vi "SEK2020v1SubVIOdometria.vi"(4 "Distância na horizontal":dbl=5.0 format="%#_13g", 6 "NXT/EV3":T1) -> (0 "Distância na vertical":dbl, 2 "NXT/EV3 2":T1)   [LabVIEW 2016]
uses:
  <vilib>/NXT/Subs/LVHSConnector.ctl
  <vilib>/NXT/LegoClasses/BrickReference/BrickReference.lvclass
  <vilib>/NXT/Block Support/NXT_OutputPort.ctl
  <vilib>/NXT/Block Support/NXT_InputPort.ctl
  <vilib>/NXT/Dual Mode Library/Sensors/EV3_Gyro_Reset.vi
  <vilib>/NXT/Dual Mode Library/Motors/ResetMotor.vi
  <vilib>/NXT/Dual Mode Library/Sensors/EV3_Gyro_Angle.vi
  <vilib>/NXT/NXTIO Xnodes/NXTIONodeSubVIs/NXTMoveMotors.vi
  <vilib>/NXT/Dual Mode Library/Motors/Rotation.vi
  <vilib>/NXT/NXTIO Xnodes/AddressXNode/NXTIOAddress.xnode
  <vilib>/NXT/NXTIO Xnodes/NXTIOXNode/NXTIO.xnode
panel:
  in  "Kp":dbl format="%#_13g"
  in  "K1":dbl
  in  "K2":dbl
  out "Dl":dbl
  out "Dr":dbl
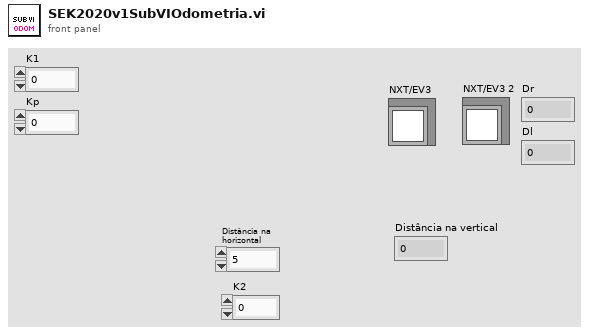
[diagram p1: front panel]
types:
  T1 = typedef "LVHSConnector.ctl" = refnum<class "BrickReference.lvclass">
  T2 = typedef "NXT_InputPort.ctl" = u32
  T3 = typedef "NXT_OutputPort.ctl" = u8
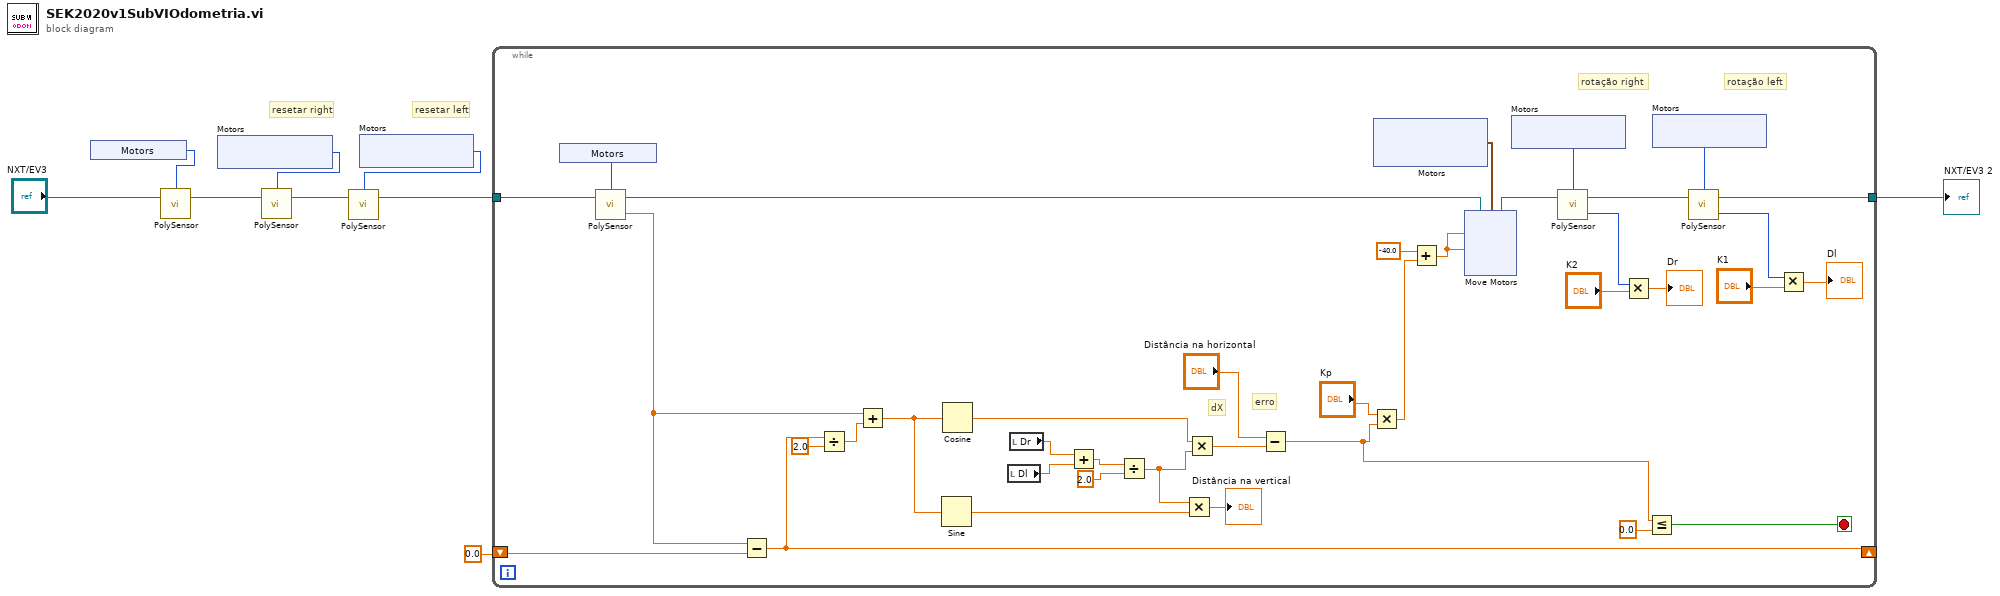
[diagram p0: block diagram]
diagram:
  # "resetar left"
  # "resetar right"
  n1 = xnode "Motors"() -> ("Sensor"=w2:T2)
  n2 = call-poly <vilib>:"PolySensor.vi"("NXT/EV3"="NXT/EV3", "Port (Port 1)"=w2) -> ("NXT/EV3"=w4:T1)  [unwired: 2 in]
  n3 = xnode "Motors"() -> ("Motor"=w8:T3)
  n4 = call-poly <vilib>:"PolySensor.vi"("NXT/EV3"=w4, "Port (All Ports)"=w8) -> ("NXT/EV3"=w7:T1)  [unwired: 2 in]
  n5 = xnode "Motors"() -> ("Motor"=w5:T3)
  n6 = call-poly <vilib>:"PolySensor.vi"("NXT/EV3"=w7, "Port (All Ports)"=w5) -> ("NXT/EV3"=w6:T1)  [unwired: 2 in]
  n7 = while {
    tunnel: w6 -> [w34]
    tunnel: [w42] -> w9
    shift-right: [w32] -> _
    shift-left: sgl 0.0 -> [w33]
    stop <- w16 stop-if-true
    # "erro"
    # "dX"
    # "rotação left"
    # "rotação right"
    n8 = xnode "Motors"() -> ("Sensor"=w44:T2)
    n9 = call-poly <vilib>:"PolySensor.vi"("NXT/EV3"=w34, "Port (Port 1)"=w44) -> ("Degrees"=w30:sgl, "NXT/EV3"=w43:T1)  [unwired: 1 in]
    n10 = Subtract(x=w30, y=w33) -> (x-y=w32:sgl)
    n11 = Divide(x=w32, y=sgl 2.0) -> (x/y=w29:sgl)
    n12 = Add(x=w30, y=w29) -> (x+y=w13:sgl)
    n13 = Sine(x=w13) -> (sin(x)=w12:sgl)
    n14 = Cosine(x=w13) -> (cos(x)=w23:sgl)
    n15 = local read "Dl"() -> (w26:dbl)
    n16 = local read "Dr"() -> (w27:dbl)
    n17 = Add(x=w27, y=w26) -> (x+y=w25:dbl)
    n18 = Divide(x=w25, y=2.0) -> (x/y=w11:dbl)
    n19 = Multiply(x=w11, y=w12) -> (x*y=→"Distância na vertical":dbl)
    n20 = Multiply(x=w23, y=w11) -> (x*y=w22:dbl)
    n21 = Subtract(x="Distância na horizontal", y=w22) -> (x-y=w15:dbl)
    n22 = Multiply(x="Kp", y=w15) -> (x*y=w19:dbl)
    n23 = xnode "Motors"() -> ("Motor"=w47:cluster{"Port":T3, "Port":T3})
    n24 = Add(x=-40.0, y=w19) -> (x+y=w17:dbl)
    n25 = xnode "Move Motors"("Power/Speed 2"=w17, "Power/Speed 1"=w17, "Motors"=w47, "NXT/EV3"=w43) -> ("NXT/EV3"=w46:T1)
    n26 = xnode "Motors"() -> ("Motor"=w41:T3)
    n27 = call-poly <vilib>:"PolySensor.vi"("NXT/EV3"=w46, "Port (Port A)"=w41) -> ("Angle of Rotation"=w39:i32, "NXT/EV3"=w45:T1)  [unwired: 1 in]
    n28 = Multiply(x=w39, y="K2") -> (x*y=→"Dr":dbl)
    n29 = Less Or Equal?(x=w15, y=0.0) -> (x <= y?=w16:bool)
    n30 = xnode "Motors"() -> ("Motor"=w40:T3)
    n31 = call-poly <vilib>:"PolySensor.vi"("NXT/EV3"=w45, "Port (Port A)"=w40) -> ("Angle of Rotation"=w37:i32, "NXT/EV3"=w42:T1)  [unwired: 1 in]
    n32 = Multiply(x=w37, y="K1") -> (x*y=→"Dl":dbl)
  }
  "NXT/EV3 2" <- w9
